vi "Chart-Move Span.vi"(8 "error in (no error)":errorcluster, 9 "Information":T1, 10 "Coords":T2, 11 "XY Graph Ref In":refnum<vi>) -> (0 "error out":errorcluster, 3 "XY Graph Ref Out":refnum<vi>)   [LabVIEW 2020]
uses:
  <vilib>/Utility/miscctls.llb/LVPoint32TypeDef.ctl
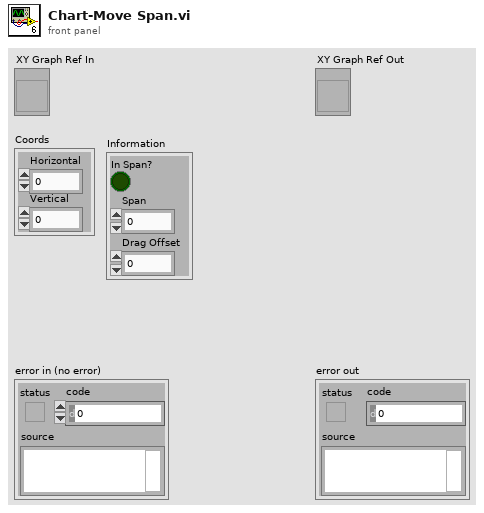
[diagram p1: front panel]
types:
  T1 = cluster{"In Span?":bool, "Span":dbl, "Drag Offset":dbl}
  T2 = typedef "LVPoint32TypeDef.ctl" = cluster{"Horizontal":i32, "Vertical":i32}
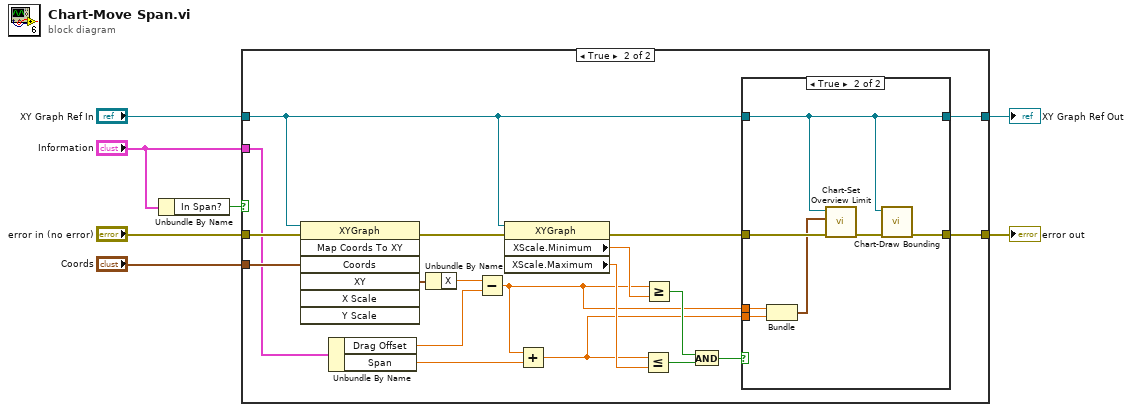
[diagram p0: block diagram]
diagram:
  n1 = Unbundle By Name("Information") -> ("In Span?"=w4:bool)
  n2 = case shown="True" w4 {
    tunnel: "error in (no error)" -> [w9 w28]
    tunnel: "Coords" -> [_ w27]
    tunnel: "XY Graph Ref In" -> [w8 w14]
    tunnel: "Information" -> [_ w25]
    tunnel: [w9 w11] -> w2
    tunnel: [w8 w10] -> w1
    frame False {
    }
    frame True {
      n3 = invoke on="Invoke Node" class="XYGraph" method="Map Coords To XY"(reference=w14, error in=w28, "Coords"=w27) -> (error out=w21:errorcluster, "XY"=w26:cluster{"X":dbl, "Y":dbl})  [unwired: 4 in, 5 out]
      n4 = Unbundle By Name(w25) -> ("Drag Offset"=w23:dbl, "Span"=w22:dbl)
      n5 = Unbundle By Name(w26) -> ("X"=w24:dbl)
      n6 = Subtract(x=w24, y=w23) -> (x-y=w13:dbl)
      n7 = property on="Property Node" class="XYGraph"(reference=w14, error in=w21) -> (error out=w15:errorcluster, "XScale.Minimum"=w20:dbl, "XScale.Maximum"=w19:dbl)  [unwired: 1 out]
      n8 = Add(x=w13, y=w22) -> (x+y=w12:dbl)
      n9 = Less Or Equal?(x=w12, y=w19) -> (x <= y?=w18:bool)
      n10 = Greater Or Equal?(x=w13, y=w20) -> (x >= y?=w17:bool)
      n11 = And(x=w17, y=w18) -> (x .and. y?=w16:bool)
      n12 = case shown="True" w16 {
        tunnel: w15 -> [w30 w37]
        tunnel: w14 -> [w29 w31]
        tunnel: w13 -> [_ w36]
        tunnel: w12 -> [_ w35]
        tunnel: [w30 w32] -> w11
        tunnel: [w29 w31] -> w10
        frame False {
        }
        frame True {
          n13 = Bundle(w36, w35) -> (w34:cluster{dbl, dbl})  [unwired: 1 in]
          n14 = call "Chart-Set Overview Limit.vi"("error in"=w37, "Limit"=w34, "Overview Refnum In"=w31) -> ("error out"=w33:errorcluster)  [unwired: 7 in, 1 out]
          n15 = call "Chart-Draw Bounding.vi"("error in (no error)"=w33, "XY Graph Ref In"=w31) -> ("error out"=w32:errorcluster)  [unwired: 8 in, 1 out]
        }
      }
    }
  }
  "error out" <- w2
  "XY Graph Ref Out" <- w1
